vi "SetSTI.vi"(8 "error in (no error)":errorcluster) -> (0 "error out":errorcluster)   [LabVIEW 2015, in "ESLSCDLL.lvlib"]
uses:
  ESLSCDLL.lvlib
  Globals.vi
  ESLSCDLL.dll
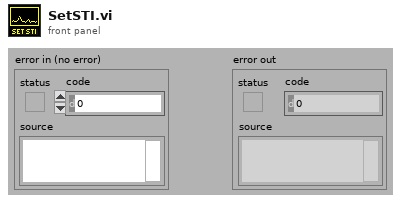
[diagram p1: front panel]
types:
  T1 = enum32{"I", "S1", "S2", "unused", "STimer", "ASL"}
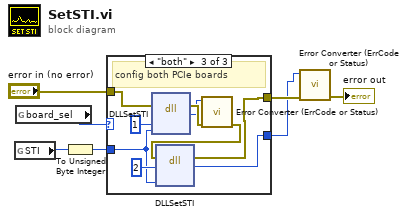
[diagram p0: block diagram]
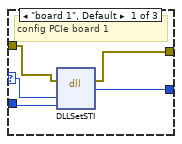
[diagram p2: hidden frame]
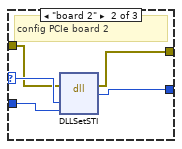
[diagram p3: hidden frame]
diagram:
  n1 = global read "Globals.vi" "STI"() -> (w2:T1)
  n2 = global read "Globals.vi" "board_sel"() -> (w3:enum32{"0", "board 1", "board 2", "both"})
  n3 = To Unsigned Byte Integer(number=w2) -> (unsigned 8bit integer=w1:u8)
  n4 = case shown="\"both\"" w3 {
    selector: w3 -> [w12 w17 _]
    tunnel: w1 -> [w11 w16 w24]
    tunnel: "error in (no error)" -> [w10 w15 w23]
    tunnel: [w9 w14 w19] -> w5
    tunnel: [w8 w13 w18] -> w4
    frame "board 1", Default {
      # "config PCIe board 1"
      n5 = dll-call lib="C:/ENTW/PCIE/LV64/board.vis/ESLSCDLL.dll" fn="DLLSetSTI" ("lwlscdll.dll:DLLRsTOREG")(error in=w10, "drv"=w12, "sti_mode"=w11) -> (error out=w9:errorcluster, "es_status_codes"=w8:i32)  [unwired: 4 in, 1 out]
    }
    frame "board 2" {
      # "config PCIe board 2"
      n6 = dll-call lib="C:/ENTW/PCIE/LV64/board.vis/ESLSCDLL.dll" fn="DLLSetSTI" ("lwlscdll.dll:DLLRsTOREG")(error in=w15, "drv"=w17, "sti_mode"=w16) -> (error out=w14:errorcluster, "return type"=w13:i32)  [unwired: 4 in, 1 out]
    }
    frame "both" {
      # "config both PCIe boards"
      n7 = dll-call lib="C:/ENTW/PCIE/LV64/board.vis/ESLSCDLL.dll" fn="DLLSetSTI" ("lwlscdll.dll:DLLRsTOREG")(error in=w23, "drv"=u32 1, "sti_mode"=w24) -> (error out=w22:errorcluster, "es_status_codes"=w21:i32)  [unwired: 4 in, 1 out]
      n8 = call "Error Converter (ErrCode or Status).vi"("error in (no error)"=w22, "error code"=w21) -> ("error out"=w20:errorcluster)  [unwired: 9 in]
      n9 = dll-call lib="C:/ENTW/PCIE/LV64/board.vis/ESLSCDLL.dll" fn="DLLSetSTI" ("lwlscdll.dll:DLLRsTOREG")(error in=w20, "drv"=u32 2, "sti_mode"=w24) -> (error out=w19:errorcluster, "es_status_codes"=w18:i32)  [unwired: 4 in, 1 out]
    }
  }
  n10 = call "Error Converter (ErrCode or Status).vi"("error in (no error)"=w5, "error code"=w4) -> ("error out"=→"error out":errorcluster)  [unwired: 9 in]
